vi "Send.vi"(7 "VolatusAPI":refnum<class "VolatusAPI.lvclass">, 10 "Value":bool, 11 "Digital Command in":refnum<class "Digital Command.lvclass">) -> (0 "error out":errorcluster)   [LabVIEW 2023, in "Volatus.lvlib" / "Digital Command.lvclass"]
uses:
  Digital Command.lvclass
  VolatusAPI/VolatusAPI.lvclass
  Digital Command.lvclass/Digital Command.ctl
  messages/CmdDigital/Class/Msg.lvclass/Msg.ctl
  VolatusAPI/VolatusAPI.lvclass/VolatusAPI.ctl
  MessageQ/MessageQ.lvclass/MessageQ.ctl
  messages/CmdDigital/Class/Msg.lvclass
  lv-vecto/Vecto/TCPMessageService/Send Message.vi
  <vilib>/Utility/error.llb/Error Cluster From Error Code.vi
  lv-protoc/LV-Proto/Message/Message.lvclass
  MessageQ/MessageQ.lvclass
  messages/CmdDigitalMultiple/Class/Msg.lvclass
  messages/CmdDigital/Data.ctl
  messages/CmdDigital/CmdDigital.lvlib
  messages/CmdDigitalMultiple/Data.ctl
  messages/CmdDigitalMultiple/CmdDigitalMultiple.lvlib
  C:/dev/volatus/mts-volatus-super/libs/lv-volatus/messages/CmdDigitalMultiple/Class/Msg.lvclass
  C:/dev/volatus/mts-volatus-super/libs/lv-protoc/LV-Proto/Message/Message.lvclass
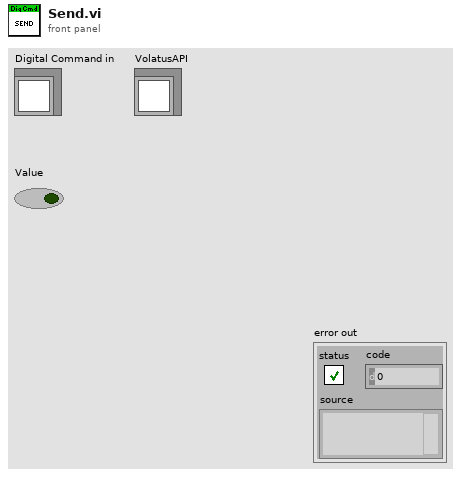
[diagram p1: front panel]
types:
  T1 = typedef "CmdDigital.lvlib/Data.ctl" = cluster{"channel":string, "value":bool}
  T2 = typedef "CmdDigitalMultiple.lvlib/Data.ctl" = cluster{"values":T1[]}
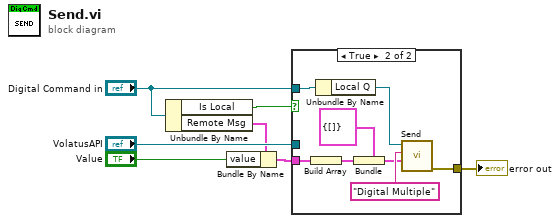
[diagram p0: block diagram]
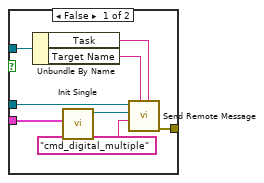
[diagram p2: hidden frame]
diagram:
  n1 = Unbundle By Name("Digital Command in") -> ("Is Local"=w7:bool, "Remote Msg"=w5:T1)
  n2 = Bundle By Name(cluster=w5, "value"="Value") -> (w3:T1)
  n3 = case shown="True" w7 {
    tunnel: "VolatusAPI" -> [w15 _]
    tunnel: w3 -> [w14 w20]
    tunnel: "Digital Command in" -> [w11 w23]
    tunnel: [w8 w19] -> w1
    frame False {
      n4 = Unbundle By Name(w11) -> ("Task"=w9:string, "Target Name"=w10:string)
      n5 = call "Init Single.vi"("value"=w14) -> ("Msg out"=w13:refnum<class "Msg.lvclass">)  [unwired: 10 in]
      n6 = call "Send Remote Message.vi"("Target Task (None)"=w9, "Target Name"=w10, "Message Type"="cmd_digital_multiple", "Message"=w13, "VolatusAPI in"=w15) -> ("error out"=w8:errorcluster)  [unwired: 5 in, 1 out]
    }
    frame True {
      n7 = Build Array(w20) -> (w17:T1[])
      n8 = Unbundle By Name(w23) -> ("Local Q"=w22:refnum<class "MessageQ.lvclass">)
      n9 = Bundle(cluster=T2 {"values"=[]} ("CmdDigitalMultiple"), "values"=w17) -> (w18:T2)
      n10 = call "Send.vi"("Data"=w18, "ID"="Digital Multiple", "MessageQ in"=w22) -> ("error out"=w19:errorcluster)  [unwired: 7 in, 1 out]
    }
  }
  "error out" <- w1
